vi "Driver Encoder Validater.vi"(8 "Progress":string, 9 "ProgressText":string) -> (2 "EndTestText":string)   [LabVIEW 2012]
panel:
  in  "EncoderGuide":dbl=3000.0
  # "What should the encoder\nbe able to get to?"
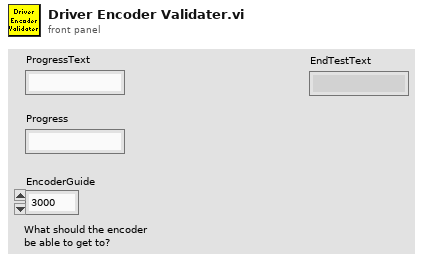
[diagram p1: front panel]
types:
  T1 = typedef "WPI_EncoderDevRef.ctl" = cluster{"DevStatus":errorcluster, "EncoderIndex":T2, "CounterIndex":T3, "DistancePerCount":dbl, "Decoding Type":T4}
  T2 = typedef "FPGA_EncoderIdx.ctl" = enum8{"Enc 0", "Enc 1", "Enc 2", "Enc 3", "Invalid"}
  T3 = typedef "FPGA_CounterCtrSystemIndex.ctl" = enum8{"Ctr 0", "Ctr 1", "Ctr 2", "Ctr 3", "Ctr 4", "Ctr 5", "Ctr 6", "Ctr 7", "Invalid"}
  T4 = typedef "WPI_EncoderType.ctl" = enum16{"1x", "2x", "4x"}
  T5 = typedef "WPI_MotorControlDeviceRef.ctl" = cluster{"DeviceStatus":errorcluster, "Type":enum16{"PWM", "CAN"}, "PWM":cluster{"Digital Module":T6, "PWM Channel":T7, "DeadBand":T8}, "CAN":cluster{"Device Number":u8, "Control Mode":T9, "Semaphore":T10, "Max Vout":dbl}, "Invert":bool, "TransformRef":T11, "InvTransformRef":T11}
  T6 = typedef "FPGA_TypedefDigitalModule.ctl" = enum16{"Digital Module 1", "Digital Module 2"}
  T7 = typedef "FPGA_DIOPWMChannel.ctl" = enum8{"PWM 1", "PWM 2", "PWM 3", "PWM 4", "PWM 5", "PWM 6", "PWM 7", "PWM 8", "PWM 9", "PWM 10", "Invalid"}
  T8 = typedef "WPI_PWMDeadband.ctl" = cluster{"Name":string, "maxPositivePwm":i32, "minPositivePwm":i32, "centerPwm":i32, "maxNegativePwm":i32, "minNegativePwm":i32, "angularRange":u16}
  T9 = typedef "WPI_CANJaguar_ControlMode.ctl" = enum8{"Percent VBus", "Current", "Speed", "Position", "Voltage"}
  T10 = typedef "Semaphore RefNum" = refnum<k1>
  T11 = typedef "WPI_PWMTransform_ConPane.ctl" = refnum<vi>
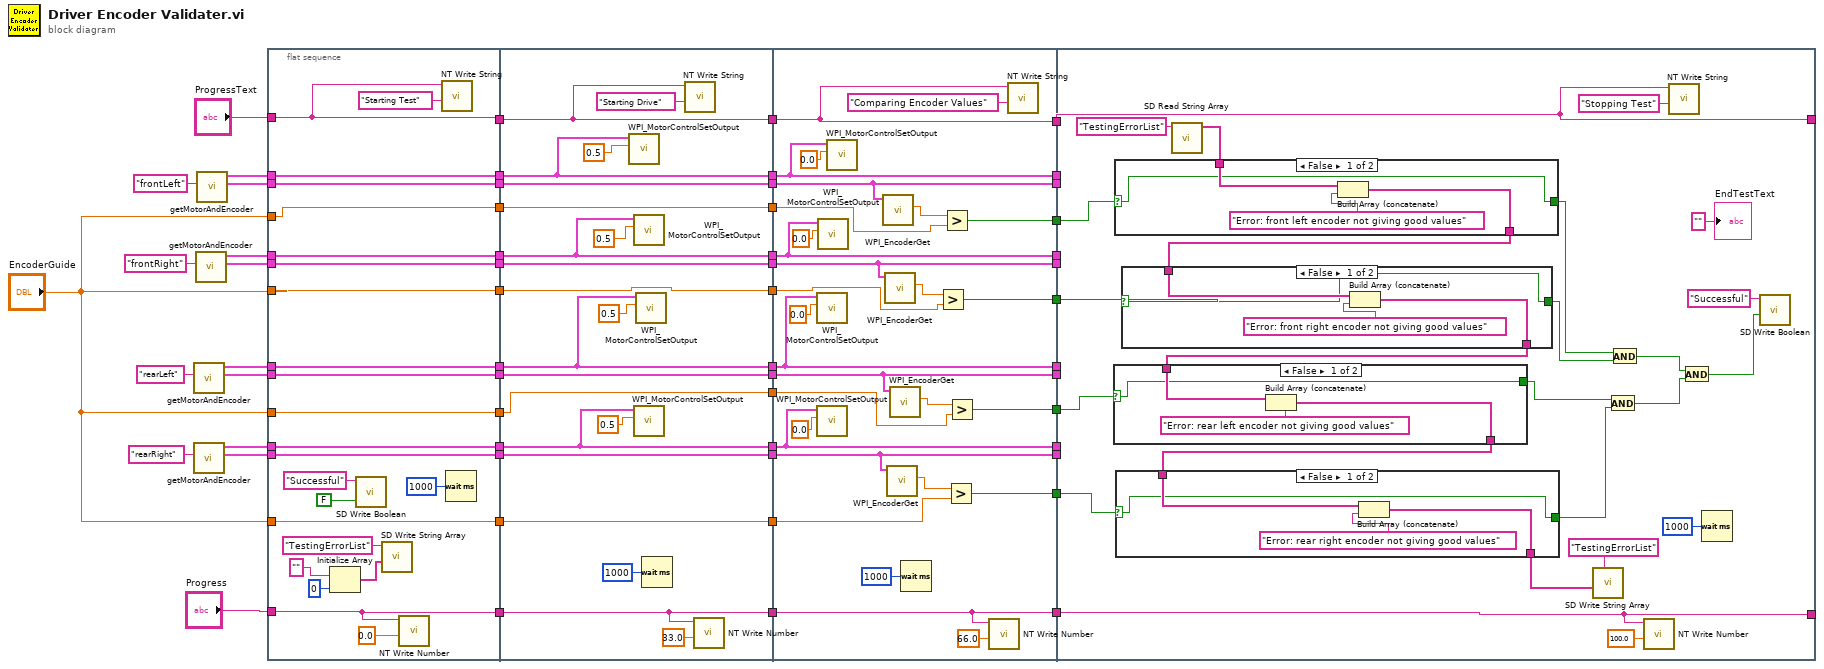
[diagram p0: block diagram]
diagram:
  n1 = call "getMotorAndEncoder.vi"("Name"="rearLeft") -> ("EncoderDevRef"=w42:T1, "MotorControlDevRef"=w44:T5)  [unwired: 8 in, 1 out]
  n2 = call "getMotorAndEncoder.vi"("Name"="rearRight") -> ("EncoderDevRef"=w38:T1, "MotorControlDevRef"=w40:T5)  [unwired: 8 in, 1 out]
  n3 = call "getMotorAndEncoder.vi"("Name"="frontRight") -> ("EncoderDevRef"=w46:T1, "MotorControlDevRef"=w48:T5)  [unwired: 8 in, 1 out]
  n4 = call "getMotorAndEncoder.vi"("Name"="frontLeft") -> ("EncoderDevRef"=w50:T1, "MotorControlDevRef"=w52:T5)  [unwired: 8 in, 1 out]
  n5 = flat-sequence {
    tunnel: "ProgressText" -> [w79]
    tunnel: "Progress" -> [w78]
    tunnel: [w79] -> w55
    tunnel: [w78] -> w54
    tunnel: [w75] -> w53
    tunnel: w52 -> [w75]
    tunnel: [w74] -> w51
    tunnel: w50 -> [w74]
    tunnel: [w73] -> w49
    tunnel: w48 -> [w73]
    tunnel: [w72] -> w47
    tunnel: w46 -> [w72]
    tunnel: [w71] -> w45
    tunnel: w44 -> [w71]
    tunnel: [w70] -> w43
    tunnel: w42 -> [w70]
    tunnel: [w69] -> w41
    tunnel: w40 -> [w69]
    tunnel: [w68] -> w39
    tunnel: w38 -> [w68]
    tunnel: "EncoderGuide" -> [w62]
    tunnel: "EncoderGuide" -> [w63]
    tunnel: "EncoderGuide" -> [w64]
    tunnel: "EncoderGuide" -> [w65]
    tunnel: [w65] -> w22
    tunnel: [w64] -> w20
    tunnel: [w63] -> w18
    tunnel: [w62] -> w15
    tunnel: w55 -> [w87]
    tunnel: w54 -> [w82]
    tunnel: w53 -> [w95]
    tunnel: w51 -> [w101]
    tunnel: w49 -> [w93]
    tunnel: w47 -> [w100]
    tunnel: w45 -> [w91]
    tunnel: w43 -> [w99]
    tunnel: w41 -> [w89]
    tunnel: w39 -> [w98]
    tunnel: [w87] -> w37
    tunnel: [w82] -> w36
    tunnel: [w101] -> w35
    tunnel: [w100] -> w34
    tunnel: [w99] -> w33
    tunnel: [w98] -> w32
    tunnel: [w95] -> w31
    tunnel: [w93] -> w30
    tunnel: [w91] -> w29
    tunnel: [w89] -> w28
    tunnel: w22 -> [w86]
    tunnel: [w86] -> w21
    tunnel: w20 -> [w85]
    tunnel: [w85] -> w19
    tunnel: w18 -> [w84]
    tunnel: [w84] -> w17
    tunnel: [w83] -> w16
    tunnel: w15 -> [w83]
    tunnel: w37 -> [w104]
    tunnel: w36 -> [w103]
    tunnel: w35 -> [w122]
    tunnel: w34 -> [w121]
    tunnel: w33 -> [w120]
    tunnel: w32 -> [w119]
    tunnel: w31 -> [w129]
    tunnel: w30 -> [w127]
    tunnel: w29 -> [w125]
    tunnel: w28 -> [w123]
    tunnel: w21 -> [w114]
    tunnel: w19 -> [w113]
    tunnel: w17 -> [w112]
    tunnel: w16 -> [w111]
    tunnel: [w104] -> w14
    tunnel: [w103] -> w13
    tunnel: [w122] -> w12
    tunnel: [w121] -> w11
    tunnel: [w120] -> w10
    tunnel: [w119] -> w9
    tunnel: [w129] -> w8
    tunnel: [w127] -> w7
    tunnel: [w125] -> w6
    tunnel: [w123] -> w5
    tunnel: [w110] -> w4
    tunnel: [w109] -> w3
    tunnel: [w108] -> w2
    tunnel: [w107] -> w1
    tunnel: w14 -> [w146]
    tunnel: w13 -> [w145]
    tunnel: w12 -> [_]
    tunnel: w11 -> [_]
    tunnel: w10 -> [_]
    tunnel: w9 -> [_]
    tunnel: w8 -> [_]
    tunnel: w7 -> [_]
    tunnel: w6 -> [_]
    tunnel: w5 -> [_]
    tunnel: w4 -> [w142]
    tunnel: w3 -> [w148]
    tunnel: w2 -> [w155]
    tunnel: w1 -> [w154]
    tunnel: [w145] -> _
    tunnel: [w146] -> _
    frame #0 {
      n6 = Initialize Array("", 0 ("dimension size")) -> (w59:string[])
      n7 = call <vilib>:"SD Write Boolean.vi"("Boolean"=FALSE, "Name"="Successful") -> ()  [unwired: 8 in, 2 out]
      n8 = call <vilib>:"SD Write String Array.vi"("String Array"=w59, "Name"="TestingErrorList") -> ()  [unwired: 8 in, 2 out]
      n9 = call <vilib>:"NT Write Number.vi"("Numeric"=0.0, "Name"=w78) -> ()  [unwired: 9 in, 1 out]
      n10 = call <vilib>:"NT Write String.vi"("String"="Starting Test", "Name"=w79) -> ()  [unwired: 9 in, 1 out]
      n11 = Wait (ms)(milliseconds to wait=u32 1000) -> ()  [unwired: 1 out]
    }
    frame #1 {
      n12 = call <vilib>:"WPI_MotorControlSetOutput.vi"("Output"=0.5, "MotorControlDevRef"=w95) -> ()  [unwired: 7 in, 3 out]
      n13 = call <vilib>:"WPI_MotorControlSetOutput.vi"("Output"=0.5, "MotorControlDevRef"=w93) -> ()  [unwired: 7 in, 3 out]
      n14 = call <vilib>:"WPI_MotorControlSetOutput.vi"("Output"=0.5, "MotorControlDevRef"=w89) -> ()  [unwired: 7 in, 3 out]
      n15 = call <vilib>:"WPI_MotorControlSetOutput.vi"("Output"=0.5, "MotorControlDevRef"=w91) -> ()  [unwired: 7 in, 3 out]
      n16 = Wait (ms)(milliseconds to wait=u32 1000) -> ()  [unwired: 1 out]
      n17 = call <vilib>:"NT Write String.vi"("String"="Starting Drive", "Name"=w87) -> ()  [unwired: 9 in, 1 out]
      n18 = call <vilib>:"NT Write Number.vi"("Numeric"=33.0, "Name"=w82) -> ()  [unwired: 9 in, 1 out]
    }
    frame #2 {
      n19 = call <vilib>:"WPI_MotorControlSetOutput.vi"("Output"=0.0, "MotorControlDevRef"=w125) -> ()  [unwired: 7 in, 3 out]
      n20 = call <vilib>:"WPI_MotorControlSetOutput.vi"("Output"=0.0, "MotorControlDevRef"=w123) -> ()  [unwired: 7 in, 3 out]
      n21 = call <vilib>:"WPI_MotorControlSetOutput.vi"("Output"=0.0, "MotorControlDevRef"=w127) -> ()  [unwired: 7 in, 3 out]
      n22 = call <vilib>:"WPI_MotorControlSetOutput.vi"("Output"=0.0, "MotorControlDevRef"=w129) -> ()  [unwired: 7 in, 3 out]
      n23 = call <vilib>:"WPI_EncoderGet.vi"("EncoderDevRef"=w122) -> ("Distance"=w118:dbl)  [unwired: 5 in, 5 out]
      n24 = call <vilib>:"WPI_EncoderGet.vi"("EncoderDevRef"=w121) -> ("Distance"=w117:dbl)  [unwired: 5 in, 5 out]
      n25 = call <vilib>:"WPI_EncoderGet.vi"("EncoderDevRef"=w119) -> ("Distance"=w115:dbl)  [unwired: 5 in, 5 out]
      n26 = call <vilib>:"WPI_EncoderGet.vi"("EncoderDevRef"=w120) -> ("Distance"=w116:dbl)  [unwired: 5 in, 5 out]
      n27 = Wait (ms)(milliseconds to wait=u32 1000) -> ()  [unwired: 1 out]
      n28 = Greater?(x=w117, y=w112) -> (0:w109:bool)
      n29 = Greater?(x=w118, y=w111) -> (0:w110:bool)
      n30 = Greater?(x=w115, y=w114) -> (0:w107:bool)
      n31 = Greater?(x=w116, y=w113) -> (0:w108:bool)
      n32 = call <vilib>:"NT Write Number.vi"("Numeric"=66.0, "Name"=w103) -> ()  [unwired: 9 in, 1 out]
      n33 = call <vilib>:"NT Write String.vi"("String"="Comparing Encoder Values", "Name"=w104) -> ()  [unwired: 9 in, 1 out]
    }
    frame #3 {
      n34 = call <vilib>:"SD Read String Array.vi"("Name"="TestingErrorList") -> ("String Array"=w140:string[])  [unwired: 9 in, 1 out]
      n35 = case shown="False" w142 {
        selector: w142 -> [w174 w178]
        tunnel: w140 -> [w176 w179]
        tunnel: [w175 w179] -> w139
        tunnel: [w174 w178] -> w135
        frame False {
          n36 = Build Array (concatenate)(w176, "Error: front left encoder not giving good values" ("String")) -> (w175:string[])
        }
        frame True {
        }
      }
      n37 = case shown="False" w148 {
        selector: w148 -> [w168 w172]
        tunnel: w139 -> [w170 w173]
        tunnel: [w169 w173] -> w138
        tunnel: [w168 w172] -> w136
        frame False {
          n38 = Build Array (concatenate)(w170, "Error: front right encoder not giving good values" ("String")) -> (w169:string[])
        }
        frame True {
        }
      }
      n39 = case shown="False" w155 {
        selector: w155 -> [w162 w167]
        tunnel: w138 -> [w164 w166]
        tunnel: [w163 w166] -> w137
        tunnel: [w162 w167] -> w134
        frame False {
          n40 = Build Array (concatenate)(w164, "Error: rear left encoder not giving good values" ("String")) -> (w163:string[])
        }
        frame True {
        }
      }
      n41 = case shown="False" w154 {
        selector: w154 -> [w156 w160]
        tunnel: w137 -> [w158 w161]
        tunnel: [w157 w161] -> w132
        tunnel: [w156 w160] -> w133
        frame False {
          n42 = Build Array (concatenate)(w158, "Error: rear right encoder not giving good values" ("String")) -> (w157:string[])
        }
        frame True {
        }
      }
      n43 = call <vilib>:"SD Write String Array.vi"("String Array"=w132, "Name"="TestingErrorList") -> ()  [unwired: 8 in, 2 out]
      n44 = And(x=w134, y=w133) -> (x .and. y?=w152:bool)
      n45 = And(x=w135, y=w136) -> (x .and. y?=w153:bool)
      n46 = call <vilib>:"NT Write Number.vi"("Numeric"=100.0, "Name"=w145) -> ()  [unwired: 9 in, 1 out]
      n47 = call <vilib>:"NT Write String.vi"("String"="Stopping Test", "Name"=w146) -> ()  [unwired: 9 in, 1 out]
      n48 = And(x=w153, y=w152) -> (x .and. y?=w150:bool)
      n49 = Wait (ms)(milliseconds to wait=u32 1000) -> ()  [unwired: 1 out]
      n50 = call <vilib>:"SD Write Boolean.vi"("Boolean"=w150, "Name"="Successful") -> ()  [unwired: 8 in, 2 out]
      "EndTestText" <- "" ("EndTestText")
    }
  }
